vi "IECMemory.ProcEvents.vi"(0 "i ref in":refnum<vi>, 5 "error in":errorcluster) -> (14 "i ref out":refnum<vi>, 19 "error out":errorcluster)   [LabVIEW 2014, in "IECMemory.lvlib"]
doc: "This method is used to define the events the object will listen to. Add your own events here."
uses:
  IECMemory.lvlib
  CS_Core/BaseProcess/BaseProcess.event definition.ctl
  CS_Core/CAEObj/CAEObj.event definition.ctl
  CS_Core/BaseProcess/BaseProcess.descriptor string definition.ctl
  CS_Core/BaseProcess/BaseProcess.lvlib
  CS_Core/CAEObj/CAEObj.lvlib
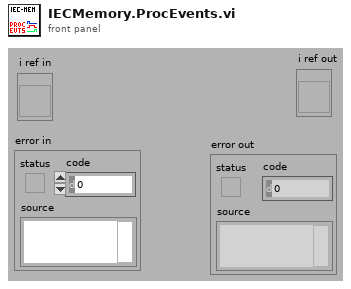
[diagram p1: front panel]
types:
  T1 = typedef "BaseProcess.lvlib/BaseProcess.event definition.ctl" = cluster{"CAEEvtDef":T2, "Data Descriptor":T3}
  T2 = typedef "CAEObj.lvlib/CAEObj.event definition.ctl" = cluster{"URL":string, "enable":bool, "ignoreResID":bool}
  T3 = typedef "BaseProcess.lvlib/BaseProcess.descriptor string definition.ctl" = string
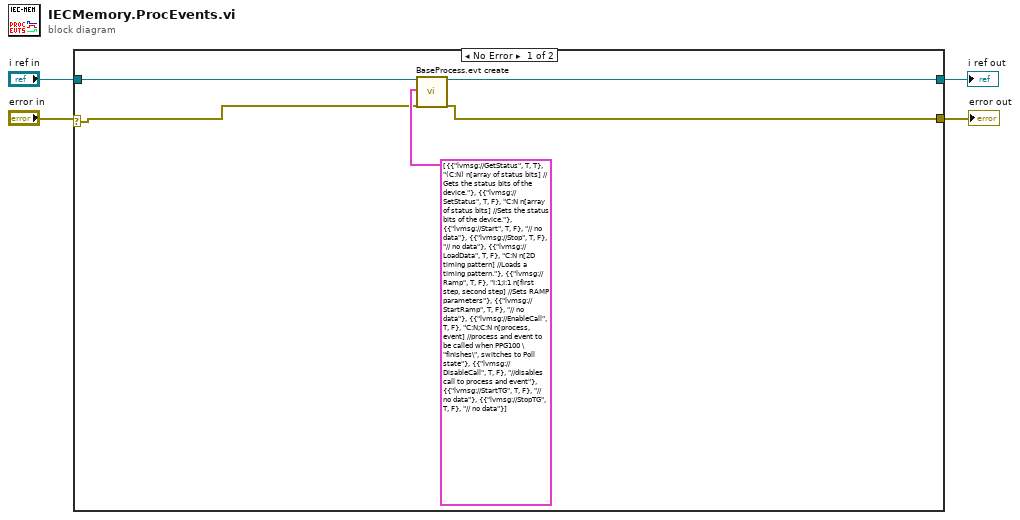
[diagram p0: block diagram]
diagram:
  n1 = case shown="No Error" "error in" {
    selector: "error in" -> [w5 w10]
    tunnel: "i ref in" -> [w9 w11]
    tunnel: [w7 w10] -> w3
    tunnel: [w6 w11] -> w2
    frame No Error {
      n2 = call "BaseProcess.evt create.vi"("i ref in"=w9, "newEvents"=T1[] [{"CAEEvtDef"={"URL"="lvmsg://GetStatus", "enable"=TRUE, "ignoreResID"=TRUE}, "Data Descriptor"="(C:N) n[array of status bits] //Gets the status bits of the device."}, {"CAEEvtDef"={"URL"="lvmsg://SetStatus", "enable"=TRUE, "ignoreResID"=FALSE}, "Data Descriptor"="C:N n[array of status bits] //Sets the status bits of the device."}, {"CAEEvtDef"={"URL"="lvmsg://Start", "enable"=TRUE, "ignoreResID"=FALSE}, "Data Descriptor"="// no data"}, {"CAEEvtDef"={"URL"="lvmsg://Stop", "enable"=TRUE, "ignoreResID"=FALSE}, "Data Descriptor"="// no data"}, {"CAEEvtDef"={"URL"="lvmsg://LoadData", "enable"=TRUE, "ignoreResID"=FALSE}, "Data Descriptor"="C:N n[2D timing pattern] //Loads a timing pattern."}, {"CAEEvtDef"={"URL"="lvmsg://Ramp", "enable"=TRUE, "ignoreResID"=FALSE}, "Data Descriptor"="I:1;I:1 n[first step, second step] //Sets RAMP parameters"}, {"CAEEvtDef"={"URL"="lvmsg://StartRamp", "enable"=TRUE, "ignoreResID"=FALSE}, "Data Descriptor"="// no data"}, {"CAEEvtDef"={"URL"="lvmsg://EnableCall", "enable"=TRUE, "ignoreResID"=FALSE}, "Data Descriptor"="C:N;C:N n[process, event] //process and event to be called when PPG100 \"finishes\", switches to Poll state"}, {"CAEEvtDef"={"URL"="lvmsg://DisableCall", "enable"=TRUE, "ignoreResID"=FALSE}, "Data Descriptor"="//disables call to process and event"}, {"CAEEvtDef"={"URL"="lvmsg://StartTG", "enable"=TRUE, "ignoreResID"=FALSE}, "Data Descriptor"="// no data"}, {"CAEEvtDef"={"URL"="lvmsg://StopTG", "enable"=TRUE, "ignoreResID"=FALSE}, "Data Descriptor"="// no data"}] ("new events"), "error in (no error)"=w5) -> ("i ref out"=w6:refnum<vi>, "error out"=w7:errorcluster)  [unwired: 13 in, 2 out]
    }
    frame Error {
    }
  }
  "i ref out" <- w2
  "error out" <- w3
